vi "SET_Path.vi"(8 "error in (no error)":errorcluster, 10 "Path":path, 11 "Icon Framework.lvclass in":refnum<class "Icon Framework.lvclass">) -> (0 "error out":errorcluster, 3 "Icon Framework.lvclass out":refnum<class "Icon Framework.lvclass">)   [LabVIEW 2020, in "Icon Framework.lvclass"]
doc: "Specify the path to the Template Layer glyph. Always pass in the fully qualified path to the glyph."
uses:
  <vilib>/LabVIEW Icon API/lv_icon/Classes/Icon Framework/Icon Framework.lvclass
  <vilib>/LabVIEW Icon API/lv_icon/Classes/Icon Framework/Icon Framework.lvclass/Icon Framework.ctl
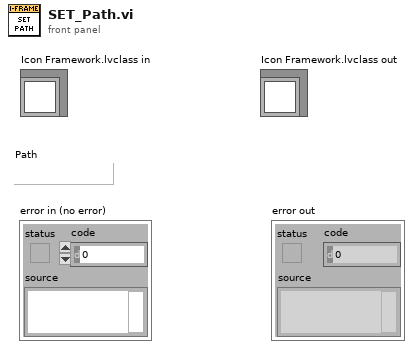
[diagram p1: front panel]
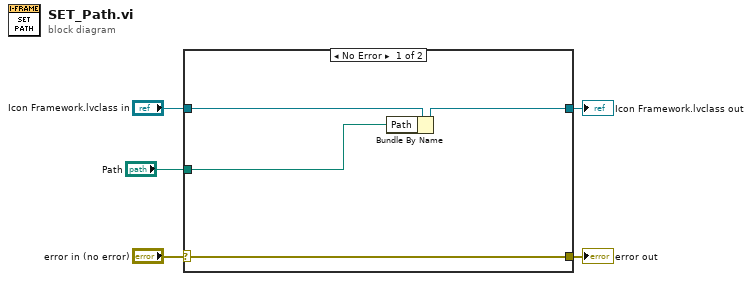
[diagram p0: block diagram]
diagram:
  n1 = case shown="No Error" "error in (no error)" {
    selector: "error in (no error)" -> [w9 w10]
    tunnel: [w9 w10] -> w4
    tunnel: [w7 w11] -> w2
    tunnel: "Icon Framework.lvclass in" -> [w8 w11]
    tunnel: "Path" -> [w6 _]
    frame No Error {
      n2 = Bundle By Name(cluster=w8, "Path"=w6) -> (w7:refnum<class "Icon Framework.lvclass">)
    }
    frame Error {
    }
  }
  "error out" <- w4
  "Icon Framework.lvclass out" <- w2
